vi "Kinematics.vi"(8 "error in (no error)":errorcluster, 11 "Data In":T1) -> (0 "error out":errorcluster, 3 "Data Out":T1)   [LabVIEW 2017]
uses:
  Type Defs/Host Data.ctl
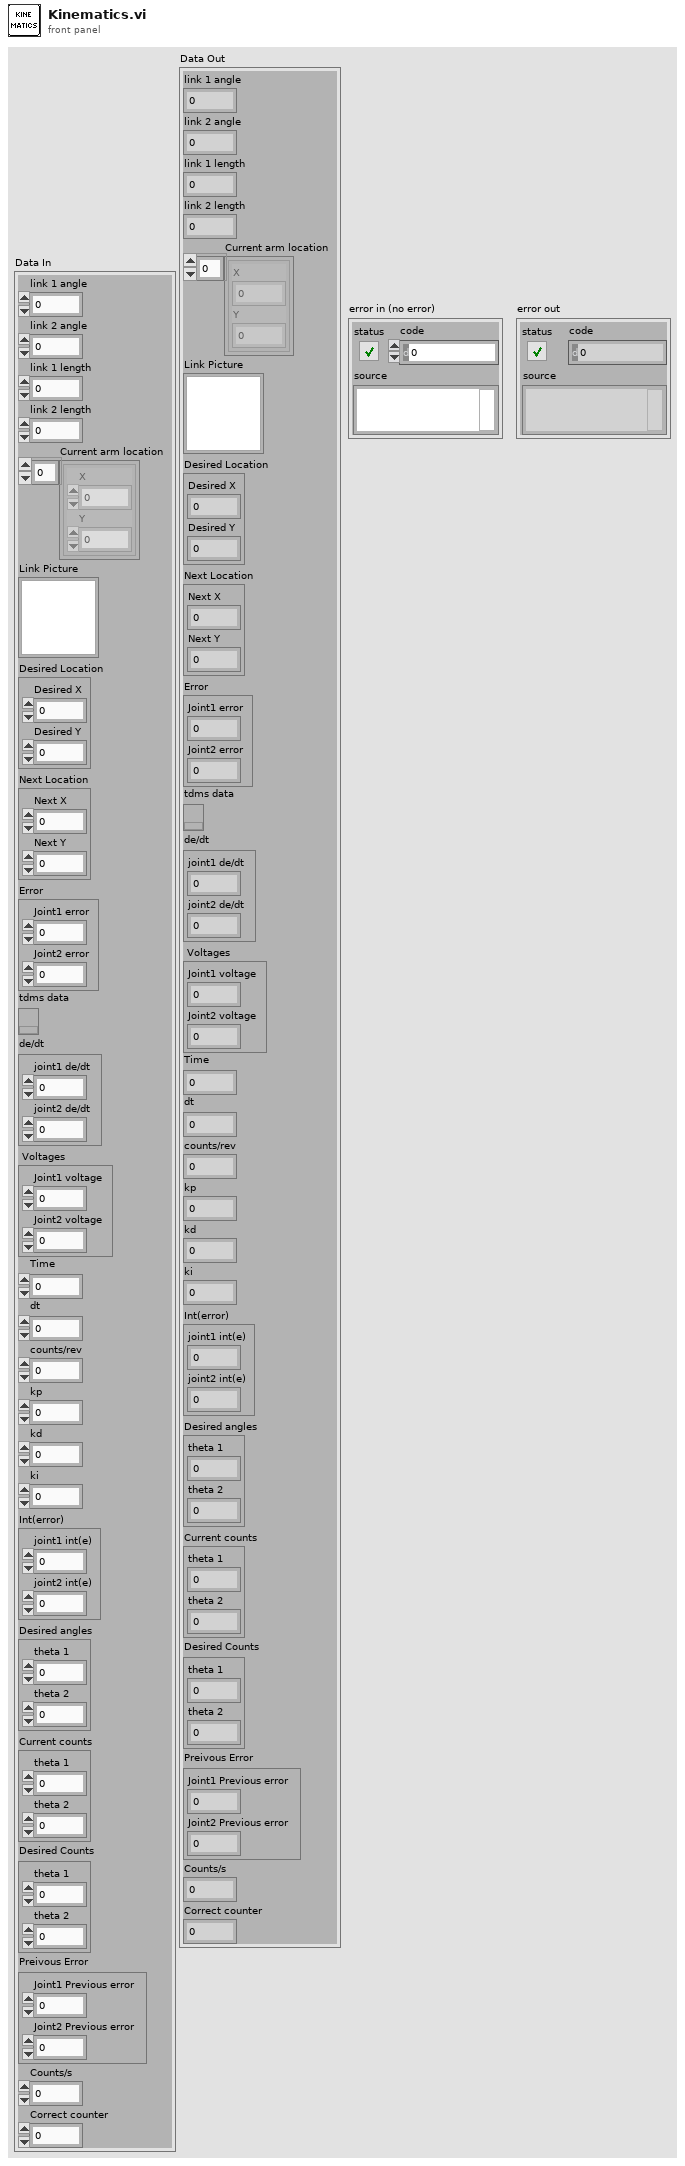
[diagram p1: front panel]
types:
  T1 = typedef "Host Data.ctl" = cluster{"link 1 angle":dbl, "link 2 angle":dbl, "link 1 length":dbl, "link 2 length":dbl, "Current arm location":cluster{"X":dbl, "Y":dbl}[], "Link Picture":picture, "Desired Location":cluster{"Desired X":dbl, "Desired Y":dbl}, "Next Location":cluster{"Next X":dbl, "Next Y":dbl}, "Error":cluster{"Joint1 error":dbl, "Joint2 error":dbl}, "tdms data":refnum<k34>, "de/dt":cluster{"joint1 de/dt":dbl, "joint2 de/dt":dbl}, "Voltages":cluster{"Joint1 voltage":dbl, "Joint2 voltage":dbl}, "Time":dbl, "dt":dbl, "counts/rev":dbl, "kp":dbl, "kd":dbl, "ki":dbl, "Int(error)":cluster{"joint1 int(e)":dbl, "joint2 int(e)":dbl}, "Desired angles":cluster{"theta 1":dbl, "theta 2":dbl}, "Current counts":cluster{"theta 1":dbl, "theta 2":dbl}, "Desired Counts":cluster{"theta 1":dbl, "theta 2":dbl}, "Preivous Error":cluster{"Joint1 Previous error":dbl, "Joint2 Previous error":dbl}, "Counts/s":dbl, "Correct counter":i32}
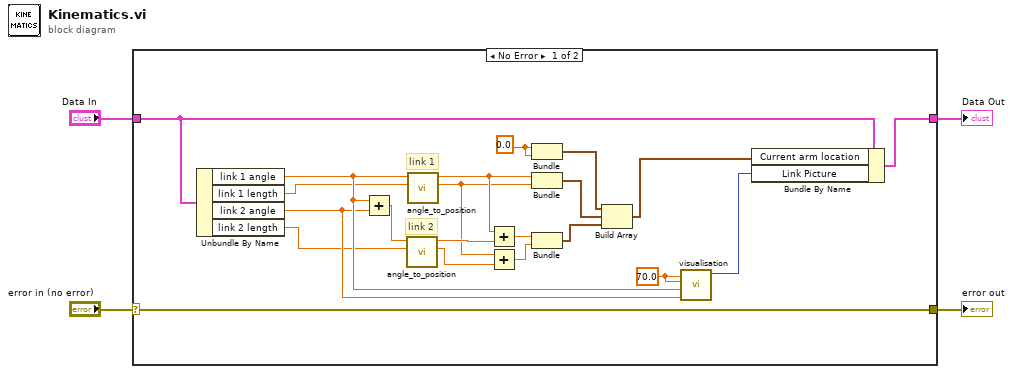
[diagram p0: block diagram]
diagram:
  n1 = case shown="No Error" "error in (no error)" {
    selector: "error in (no error)" -> [w6 w26]
    tunnel: "Data In" -> [w8 w27]
    tunnel: [w7 w27] -> w3
    tunnel: [w6 w26] -> w1
    frame No Error {
      w16 = 0.0
      w24 = 70.0 ("Length A")
      # "link 2"
      # "link 1"
      n2 = Unbundle By Name(w8) -> ("link 1 angle"=w13:dbl, "link 1 length"=w12:dbl, "link 2 angle"=w11:dbl, "link 2 length"=w10:dbl)
      n3 = Add(x=w13, y=w11) -> (x+y=w15:dbl)
      n4 = call "angle_to_position.vi"("arm length"=w10, "angle"=w15) -> ("y position"=w22:dbl, "x position"=w23:dbl)  [unwired: 8 in]
      n5 = call "angle_to_position.vi"("arm length"=w12, "angle"=w13) -> ("y position"=w20:dbl, "x position"=w21:dbl)  [unwired: 8 in]
      n6 = Add(x=w21, y=w23) -> (x+y=w14:dbl)
      n7 = Add(x=w20, y=w22) -> (x+y=w5:dbl)
      n8 = Bundle(w16, w16) -> (w17:cluster{dbl, dbl})  [unwired: 1 in]
      n9 = Bundle("x position"=w21, "y position"=w20) -> (w19:cluster{"x position":dbl, "y position":dbl})  [unwired: 1 in]
      n10 = Bundle(w14, w5) -> (w18:cluster{dbl, dbl})  [unwired: 1 in]
      n11 = Build Array(w17, w19, w18) -> (w9:cluster{"x position":dbl, "y position":dbl}[])
      n12 = call "visualisation.vi"("Joint B"=w11, "Joint A"=w13, "Length B"=w24, "Length A"=w24) -> ("Picture"=w25:picture)  [unwired: 7 in]
      n13 = Bundle By Name(cluster=w8, "Current arm location"=w9, "Link Picture"=w25) -> (w7:T1)
    }
    frame Error {
    }
  }
  "Data Out" <- w3
  "error out" <- w1
